vi "Find Peak (SubVI).vi"(8 "Last Peak Distance":u16, 9 "Index":i16, 10 "Max Angle":fxp<+/-,16,3> format="%.29g", 11 "Angle":fxp<+/-,16,3> format="%.14g") -> (3 "Peak?":bool)   [LabVIEW 2015]
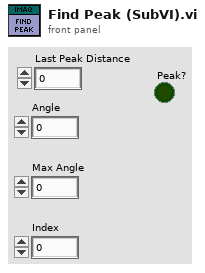
[diagram p1: front panel]
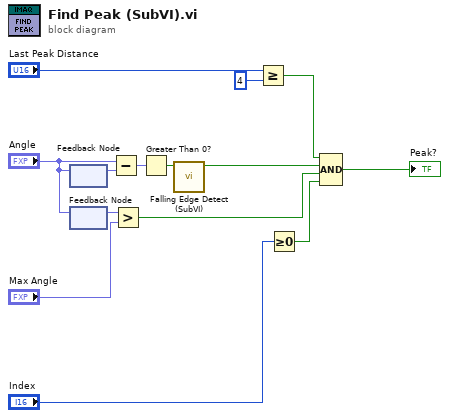
[diagram p0: block diagram]
diagram:
  n1 = feedback #1() -> (w6:fxp<+/-,16,3>)  [unwired: 1 in]
  n2 = feedback-in #1("Angle") -> ()
  n3 = feedback #2() -> (w13:fxp<+/-,16,3>)  [unwired: 1 in]
  n4 = feedback-in #2("Angle") -> ()
  n5 = Subtract(x="Angle", y=w6) -> (x-y=w7:fxp<+/-,17,4>)
  n6 = Greater?(x=w13, y="Max Angle") -> (0:w9:bool)
  n7 = Greater Than 0?(x=w7) -> (x > 0?=w8:bool)
  n8 = call "Falling Edge Detect (SubVI).vi"("Input"=w8) -> ("Falling Edge?"=w11:bool)  [unwired: 10 in]
  n9 = Greater Or Equal?(x="Last Peak Distance", y=u16 4 ("x")) -> (x >= y?=w2:bool)
  n10 = Greater Or Equal To 0?(x="Index") -> (x >= 0?=w10:bool)
  n11 = Compound Arithmetic op=AND(w2, w11, w9, w10) -> (→"Peak?":bool)
